vi "Get Sensor Values.vi"(14 "Ref_Drive 1R":T1, 15 "Ref_Drive 2R":T1, 16 "Ref_Drive 6R":T1, 17 "Ref_Drive 3L":T1, 18 "Ref_Drive 4L":T1, 19 "Ref_Drive 5L":T1) -> ()   [LabVIEW 2018]
uses:
  <vilib>/Rock Robotics/WPI/MotorControl/WPI_MotorControlDeviceRef.ctl
  <vilib>/Rock Robotics/WPI/MotorControl/WPI_MotorControlType.ctl
  <vilib>/Rock Robotics/SystemInterfaces/DIO/FPGA_DIOPWMChannel.ctl
  <vilib>/Rock Robotics/WPI/PWM/WPI_PWMDeadband.ctl
  <vilib>/Rock Robotics/SystemInterfaces/DIO/FPGA_DIOChannel.ctl
  OneDrive/Desktop/2019 FRC Summer Rebuild/2019_Robot_Project/2019 Summer Rebuild/Sensor Readings.vi
  OneDrive/Desktop/2019 FRC Summer Rebuild/2019_Robot_Project/2019 Summer Rebuild/CurrentMonitoring.vi
  OneDrive/Desktop/2019 FRC Summer Rebuild/2019_Robot_Project/2019 Summer Rebuild/Robot States.vi
panel:
  out "Drive Encoder Velocities":cluster{dbl, dbl}
  in  "Plot Drive Encoder Data":bool
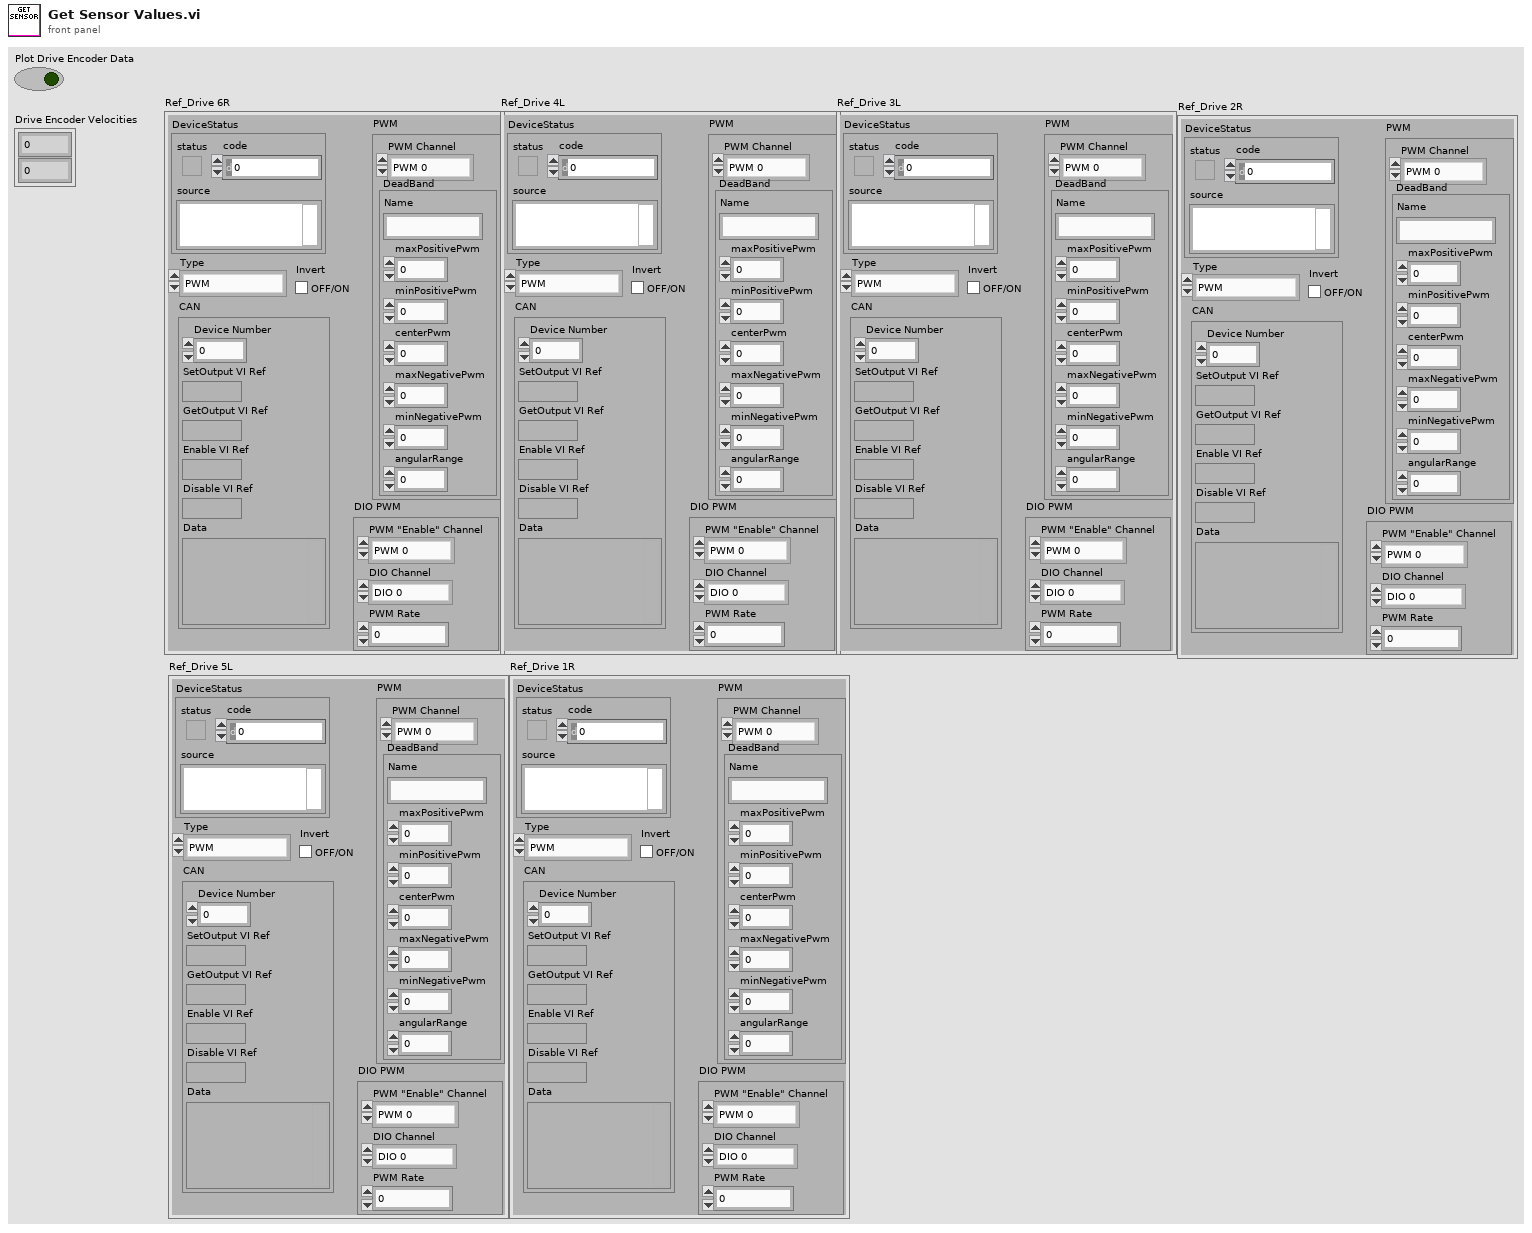
[diagram p1: front panel]
types:
  T1 = typedef "WPI_MotorControlDeviceRef.ctl" = cluster{"DeviceStatus":errorcluster, "Type":T2, "PWM":cluster{"PWM Channel":T3, "DeadBand":T4}, "CAN":cluster{"Device Number":u8, "SetOutput VI Ref":variant, "GetOutput VI Ref":variant, "Enable VI Ref":variant, "Disable VI Ref":variant, "Data":variant}, "Invert":bool, "DIO PWM":cluster{"PWM \"Enable\" Channel":T3, "DIOChannel":T5, "PWM Rate":dbl}}
  T2 = typedef "WPI_MotorControlType.ctl" = enum16{"PWM", "CAN", "DIO PWM"}
  T3 = typedef "FPGA_DIOPWMChannel.ctl" = enum8{"PWM 0", "PWM 1", "PWM 2", "PWM 3", "PWM 4", "PWM 5", "PWM 6", "PWM 7", "PWM 8", "PWM 9", "PWM MXP 0", "PWM MXP 1", "PWM MXP 2", "PWM MXP 3", "PWM MXP 4", "PWM MXP 5", "PWM MXP 6", "PWM MXP 7", "PWM MXP 8", "PWM MXP 9", "Invalid"}
  T4 = typedef "WPI_PWMDeadband.ctl" = cluster{"Name":string, "maxPositivePwm":i32, "minPositivePwm":i32, "centerPwm":i32, "maxNegativePwm":i32, "minNegativePwm":i32, "angularRange":u16}
  T5 = typedef "FPGA_DIOChannel.ctl" = enum8{"DIO 0", "DIO 1", "DIO 2", "DIO 3", "DIO 4", "DIO 5", "DIO 6", "DIO 7", "DIO 8", "DIO 9", "DIO MXP 0", "DIO MXP 1", "DIO MXP 2", "DIO MXP 3", "DIO MXP 4", "DIO MXP 5", "DIO MXP 6", "DIO MXP 7", "DIO MXP 8", "DIO MXP 9", "DIO MXP 10", "DIO MXP 11", "DIO MXP 12", "DIO MXP 13", "DIO MXP 14", "DIO MXP 15", "SPI Port CS1", "SPI Port CS2", "SPI Port CS3", "SPI Port MISO", "SPI Port MOSI", "Invalid"}
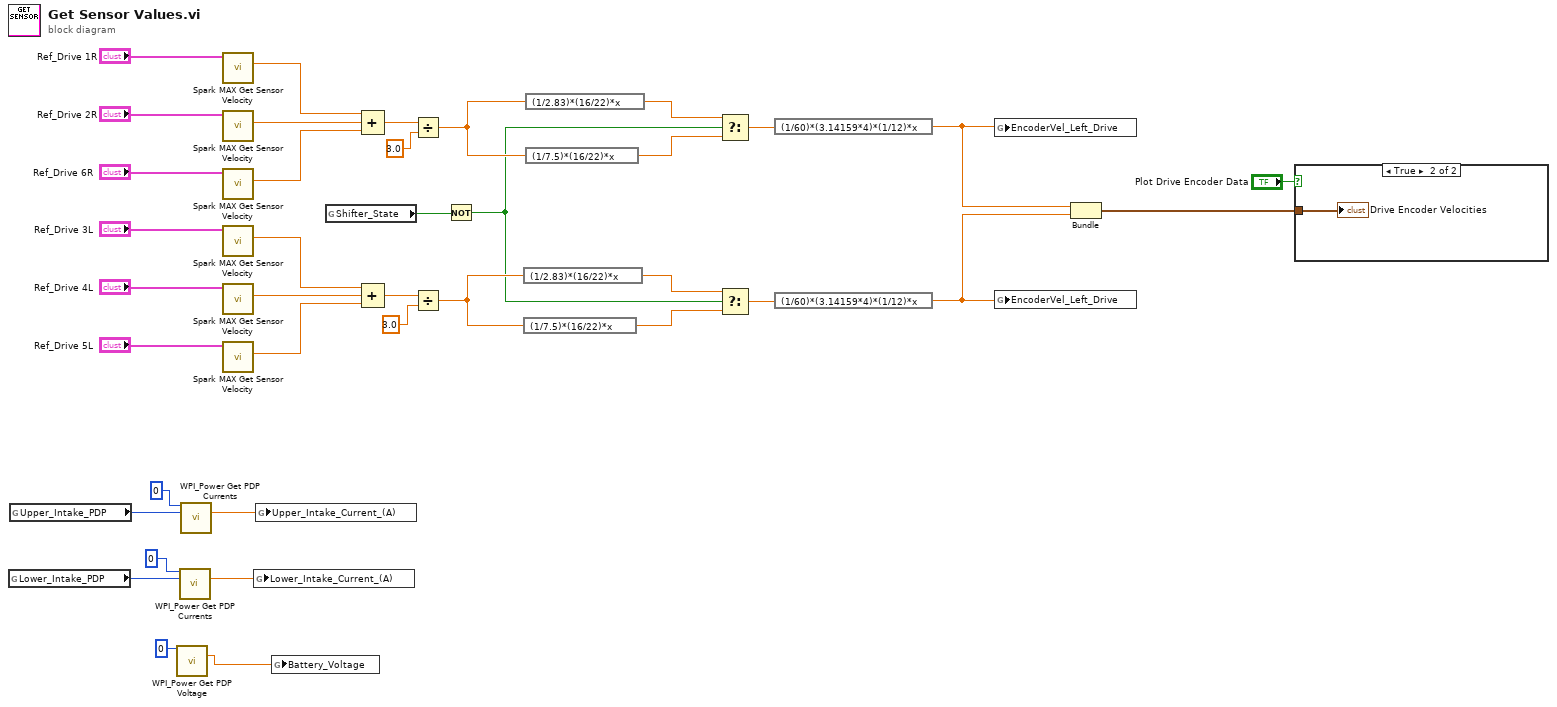
[diagram p0: block diagram]
diagram:
  n1 = global read "CurrentMonitoring.vi" "Lower_Intake_PDP"() -> (w36:i8)
  n2 = global read "CurrentMonitoring.vi" "Upper_Intake_PDP"() -> (w37:i8)
  n3 = call <vilib>:"WPI_Power Get PDP Voltage.vi"("Power Distribution Panel (0)"=u8 0) -> ("voltage (V)"=w32:dbl)  [unwired: 13 in, 1 out]
  n4 = call <vilib>:"WPI_Power Get PDP Currents.vi"("Power Distribution Panel (0)"=u8 0, "PDP Channel"=w36) -> ("current (A)"=w38:dbl)  [unwired: 11 in, 2 out]
  n5 = call <vilib>:"WPI_Power Get PDP Currents.vi"("Power Distribution Panel (0)"=u8 0, "PDP Channel"=w37) -> ("current (A)"=w33:dbl)  [unwired: 11 in, 2 out]
  n6 = call <vilib>:"Spark MAX Get Sensor Velocity.vi"("MotorControlDevRef in"="Ref_Drive 1R") -> ("Sensor Velocity"=w24:dbl)  [unwired: 7 in, 3 out]
  n7 = call <vilib>:"Spark MAX Get Sensor Velocity.vi"("MotorControlDevRef in"="Ref_Drive 2R") -> ("Sensor Velocity"=w23:dbl)  [unwired: 7 in, 3 out]
  n8 = call <vilib>:"Spark MAX Get Sensor Velocity.vi"("MotorControlDevRef in"="Ref_Drive 6R") -> ("Sensor Velocity"=w22:dbl)  [unwired: 7 in, 3 out]
  n9 = call <vilib>:"Spark MAX Get Sensor Velocity.vi"("MotorControlDevRef in"="Ref_Drive 3L") -> ("Sensor Velocity"=w21:dbl)  [unwired: 7 in, 3 out]
  n10 = call <vilib>:"Spark MAX Get Sensor Velocity.vi"("MotorControlDevRef in"="Ref_Drive 4L") -> ("Sensor Velocity"=w20:dbl)  [unwired: 7 in, 3 out]
  n11 = call <vilib>:"Spark MAX Get Sensor Velocity.vi"("MotorControlDevRef in"="Ref_Drive 5L") -> ("Sensor Velocity"=w19:dbl)  [unwired: 7 in, 3 out]
  n12 = global write "Sensor Readings.vi" "Lower_Intake_Current_(A)"(w38) -> ()
  n13 = global write "Sensor Readings.vi" "Upper_Intake_Current_(A)"(w33) -> ()
  n14 = global write "Sensor Readings.vi" "Battery_Voltage"(w32) -> ()
  n15 = global read "Robot States.vi" "Shifter_State"() -> (w14:bool)
  n16 = Compound Arithmetic op=ADD(w24, w23, w22) -> (w16:dbl)
  n17 = Compound Arithmetic op=ADD(w21, w20, w19) -> (w15:dbl)
  n18 = Divide(x=w16, y=3.0) -> (x/y=w12:dbl)
  n19 = Divide(x=w15, y=3.0) -> (x/y=w13:dbl)
  n20 = Not(x=w14) -> (.not. x?=w7:bool)
  n21 = expression code="(1/2.83)*(16/22)*x"(w13) -> (w9:dbl)
  n22 = expression code="(1/7.5)*(16/22)*x"(w13) -> (w8:dbl)
  n23 = expression code="(1/2.83)*(16/22)*x"(w12) -> (w11:dbl)
  n24 = expression code="(1/7.5)*(16/22)*x"(w12) -> (w10:dbl)
  n25 = Select(t=w11, s=w7, f=w10) -> (s? t:f=w6:dbl)
  n26 = Select(t=w9, s=w7, f=w8) -> (s? t:f=w5:dbl)
  n27 = expression code="(1/60)*(3.14159*4)*(1/12)*x"(w6) -> (w4:dbl)
  n28 = expression code="(1/60)*(3.14159*4)*(1/12)*x"(w5) -> (w3:dbl)
  n29 = global write "Sensor Readings.vi" "EncoderVel_Left_Drive"(w4) -> ()
  n30 = global write "Sensor Readings.vi" "EncoderVel_Left_Drive"(w3) -> ()
  n31 = Bundle(w4, w3) -> (w1:cluster{dbl, dbl})  [unwired: 1 in]
  n32 = case shown="True" "Plot Drive Encoder Data" {
    tunnel: w1 -> [_ w39]
    frame False {
    }
    frame True {
      "Drive Encoder Velocities" <- w39
    }
  }
